vi "CUST Get Phasor Configuration.vi"(9 "phasorIndex":i32, 10 "pmuIndex":i32, 11 "pseudoPdcId":i32) -> (0 "function return":i32, 2 "name out":string, 3 "phasorCfg out":T1)   [LabVIEW 2013, in "C37118-DLL.lvlib"]
doc: "STRONGRIDIEEEC37118DLL_API int __cdecl getPhasorConfig(phasorConfig *phasorCfg, int32_t pseudoPdcId, int32_t pmuIndex, int32_t phasorIndex);"
uses:
  C37118-DLL.lvlib
  builds/StrongridDLL/StrongridDLL.dll
panel:
  in  "phasorCfg":T1
  in  "name":string
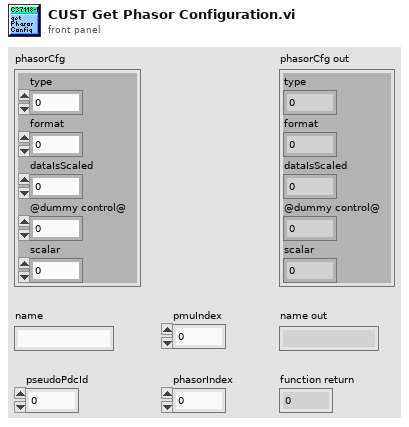
[diagram p1: front panel]
types:
  T1 = cluster{"type":u8, "format":u8, "dataIsScaled":u8, "@dummy control@":i8, "scalar":sgl}
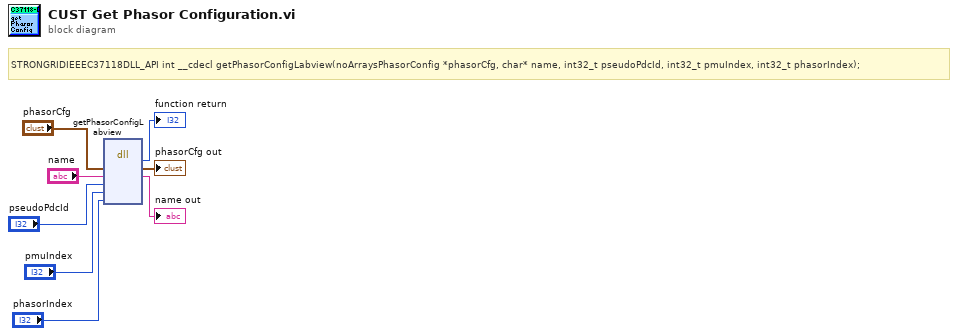
[diagram p0: block diagram]
diagram:
  # "STRONGRIDIEEEC37118DLL_API int __cdecl getPhasorConfigLabview(noArraysPhasorConfig *phasorCfg, char* name, int32_t pseudoPdcId, int32_t pmuIndex, int32_t phasorIndex);"
  n1 = dll-call lib="C:/dev/OSS/S3DK/builds/StrongridDLL/StrongridDLL.*" fn="getPhasorConfigLabview"("phasorCfg"="phasorCfg", "name"="name", "pseudoPdcId"="pseudoPdcId", "pmuIndex"="pmuIndex", "phasorIndex"="phasorIndex") -> (→"function return":i32, "phasorCfg"=→"phasorCfg out":T1, "name"=→"name out":string)  [unwired: 6 in, 2 out]
